vi "Set Bitfile Path.vi"(8 "error in (no error)":errorcluster, 10 "Bitfile Path in":path, 11 "Device Ref in":T1 format="%.0x") -> (0 "error out":errorcluster, 3 "Device Ref out":T1 format="%.0x")   [LabVIEW 2013, in "PWM System Explorer.lvlib"]
uses:
  PWM System Explorer.lvlib
  <vilib>/NI Veristand/Custom Device API/Custom Device Item Ref.ctl
  <vilib>/NI Veristand/Custom Device API/Dependent File Optional Info.ctl
  Shared/Constants.vi
  <vilib>/NI Veristand/Custom Device Offline API/Custom Device Offline API.lvlib
  <vilib>/NI Veristand/Custom Device API/Custom Device API.lvlib
  Shared/PWM Shared.lvlib
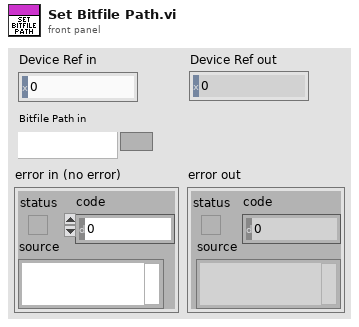
[diagram p1: front panel]
types:
  T1 = typedef "Custom Device API.lvlib/Custom Device Item Ref.ctl" = u64
  T2 = typedef "Custom Device API.lvlib/Dependent File Optional Info.ctl" = cluster{"Version":string, "RTDestination":path, "ForceDownload":bool, "SupportedTarget":string, "MD5":string}
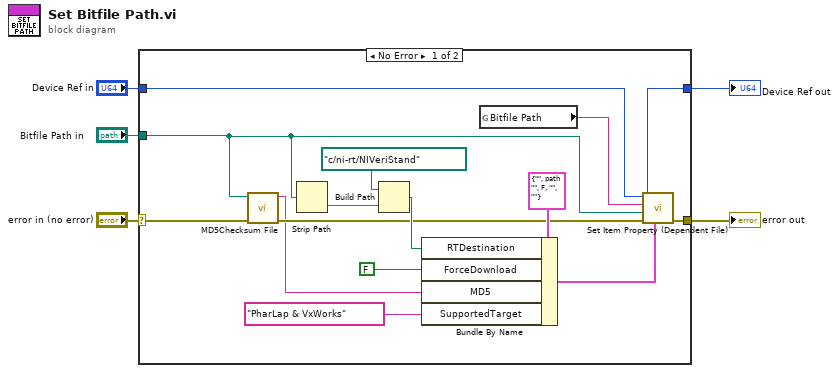
[diagram p0: block diagram]
diagram:
  n1 = case shown="No Error" "error in (no error)" {
    selector: "error in (no error)" -> [w11 w22]
    tunnel: [w20 w21] -> w5
    tunnel: "Device Ref in" -> [w19 w21]
    tunnel: "Bitfile Path in" -> [w7 _]
    tunnel: [w12 w22] -> w2
    frame No Error {
      n2 = call <vilib>:"MD5Checksum File.vi"("error in (no error)"=w11, "Path"=w7) -> ("error out"=w10:errorcluster, "MD5 message-digest"=w9:string)  [unwired: 8 in]
      n3 = Strip Path(path=w7) -> (name=w16:string)  [unwired: 1 out]
      n4 = Build Path(base path=path "c:/ni-rt/NIVeriStand", name or relative path=w16) -> (appended path=w17:path)
      n5 = Bundle By Name(cluster=T2 {"Version"="", "RTDestination"=path "", "ForceDownload"=FALSE, "SupportedTarget"="", "MD5"=""} ("OptionalInfo"), "RTDestination"=w17, "ForceDownload"=FALSE, "MD5"=w9, "SupportedTarget"="PharLap & VxWorks") -> (w18:T2)
      n6 = global read "Constants.vi" "Bitfile Path"() -> (w6:string)
      n7 = call <vilib>:"Set Item Property (Dependent File).vi"("OptionalInfo"=w18, "error in (no error)"=w10, "Path"=w7, "Property Name"=w6, "Item Ref in"=w19) -> ("error out"=w12:errorcluster, "Item Ref out"=w20:T1)  [unwired: 4 in, 1 out]
    }
    frame Error {
    }
  }
  "Device Ref out" <- w5
  "error out" <- w2
